vi "Digital Output Single Write.vi"() -> ()   [LabVIEW 2009, in "MicroDAQ.lvlib"]
uses:
  <instrlib>/MicroDAQ/MicroDAQ.lvlib
  <instrlib>/MicroDAQ/Tools/Digital IO channels.ctl
  <instrlib>/MicroDAQ/Channel/Digital output/Write NPort 1Samp 1D Boolean.vi
  <instrlib>/MicroDAQ/Channel/Digital output/Digital output.lvclass
panel:
  in  "data":u8[](array[numeric])=[1] format="%08b"
  in  "Lines":T1[](array[typedef])=[2] items=["DIO1...8"=1, "DIO9...16"=2, "DIO17...24"=3, "DIO25...32"=4]
  in  "IP address":string="10.10.1.1"
  # "Device settings"
  # "Channel Settings"
  # "Configure Output"
  # "The number of elements in data array must equal the number of configured Ports."
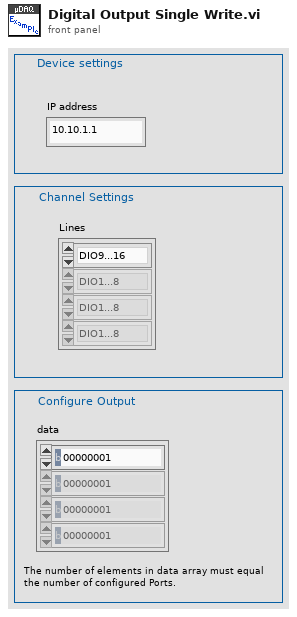
[diagram p1: front panel]
types:
  T1 = typedef "MicroDAQ.lvlib/Digital IO channels.ctl" = u16
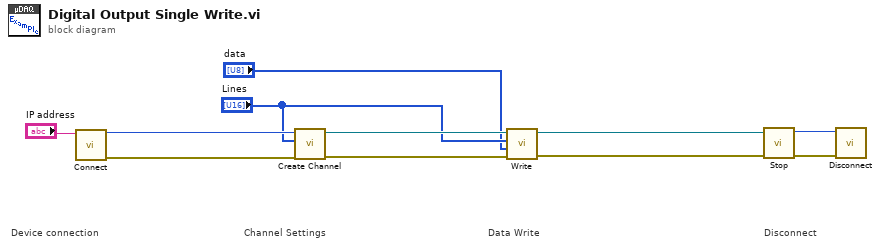
[diagram p0: block diagram]
diagram:
  # "Disconnect"
  # "Data Write"
  # "Channel Settings"
  # "Device connection"
  n1 = call <instrlib>:"Connect.vi"("IP address"="IP address") -> ("error out"=w11:errorcluster, "connection ID"=w10:i32)  [unwired: 9 in]
  n2 = call-poly <instrlib>:"Create Channel.vi"("error in (no error)"=w11, "Lines"="Lines", "Connection ID"=w10) -> ("error out"=w6:errorcluster, "MicroDAQ.lvlib:Digital output.lvclass"=w5:refnum<class "Digital output.lvclass">)  [unwired: 7 in]
  n3 = call-poly <instrlib>:"Write.vi"("error in (no error)"=w6, "values"="data", "Ports (Banks)"="Lines", "MicroDAQ.lvlib:Digital output.lvclass"=w5) -> ("error out"=w3:errorcluster, "MicroDAQ.lvlib:Digital output.lvclass out"=w4:refnum<class "Digital output.lvclass">)  [unwired: 6 in]
  n4 = call-dynamic "Stop.vi"("error in (no error)"=w3, "Task in"=w4) -> ("error out"=w8:errorcluster, "connection ID"=w7:i32)  [unwired: 8 in]
  n5 = call <instrlib>:"Disconnect.vi"("error in (no error)"=w8, "connection ID"=w7) -> ()  [unwired: 9 in, 1 out]
